vi "ProcessTemplate (Minimal).vi"   [LabVIEW 2021]
uses:
  SMO/SMO.lvclass
types:
  T1 = typedef "smo.lvlib/SMO.lvclass/Protected Events.ctl" = cluster{"StopProcesses":refnum<user-event>, "AbortProcesses":refnum<user-event>, "Config Changed":refnum<user-event>, "Dependency":refnum<user-event>}
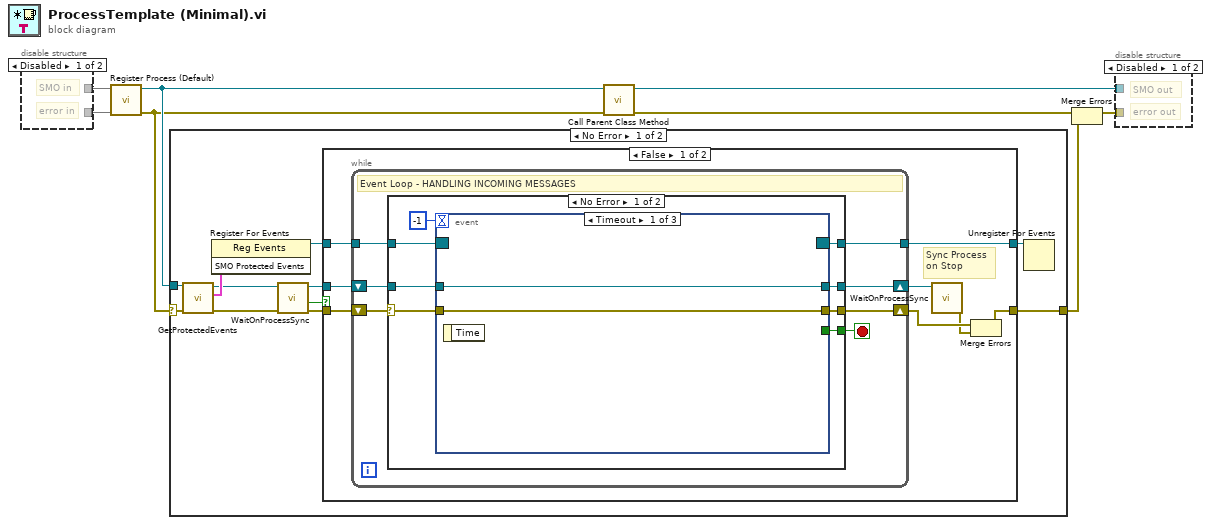
[diagram p0: block diagram]
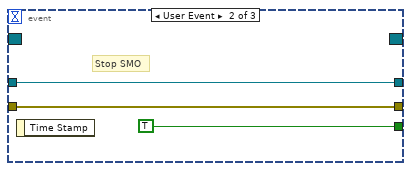
[diagram p4: hidden frame]
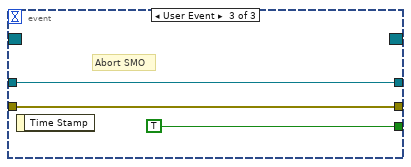
[diagram p5: hidden frame]
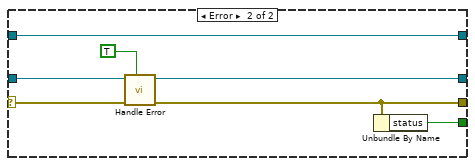
[diagram p6: hidden frame]
diagram:
  n1 = disable-structure shown="Disabled" {
    disable-tunnel: [_ _] -> w2
    disable-tunnel: [_ _] -> w1
    frame Disabled {
      # "error in"
      # "SMO in"
    }
    frame Enabled {
    }
  }
  n2 = call "Register Process (Default).vi"("error in (no error)"=w1, "SMO"=w2) -> ("error out"=w3:errorcluster, "SelfRef"=w4:refnum<class "SMO.lvclass">)  [unwired: 8 in]
  n3 = case shown="No Error" w3 {
    selector: w3 -> [w15 w60]
    tunnel: w4 -> [w18 _]
    tunnel: [w11 w60] -> w7
    frame No Error {
      n4 = call "GetProtectedEvents.vi"("error in (no error)"=w15, "SMO"=w18) -> ("error out"=w16:errorcluster, "SMO Protected Events"=w19:T1, "SMO out"=w17:refnum<class "SMO.lvclass">)  [unwired: 7 in]
      n5 = register-events(w19) -> (reference out=w9:refnum<event-registration>)  [unwired: 2 in, 1 out]
      n6 = call "WaitOnProcessSync.vi"("error in (no error)"=w16, "SMO"=w17) -> ("error out"=w13:errorcluster, "Don't run?"=w12:bool, "SMO out"=w14:refnum<class "SMO.lvclass">)  [unwired: 7 in]
      n7 = case shown="False" w12 {
        tunnel: w13 -> [w23 w58]
        tunnel: w14 -> [w25 _]
        tunnel: w9 -> [w27 w59]
        tunnel: [w20 w58] -> w11
        tunnel: [w26 w59] -> w10
        frame False {
          # "Sync Process\non Stop"
          n8 = while {
            tunnel: w27 -> [w34]
            tunnel: [w33] -> w26
            shift-right: [w30] -> w24
            shift-left: w25 -> [w31]
            shift-right: [w29] -> w22
            shift-left: w23 -> [w28]
            stop <- w32 stop-if-true
            # "Event Loop - HANDLING INCOMING MESSAGES"
            n9 = case shown="No Error" w28 {
              selector: w28 -> [w35 w55]
              tunnel: w34 -> [w41 w57]
              tunnel: [w40 w57] -> w33
              tunnel: [w39 w51] -> w32
              tunnel: w31 -> [w38 w54]
              tunnel: [w37 w53] -> w30
              tunnel: [w36 w52] -> w29
              frame No Error {
                n10 = event shown="[0] Timeout" {
                  selector: w41 -> [_ _ _]
                  dyn-events: [_ _ _] -> w40
                  timeout: -1 -> [_ _ _]
                  tunnel: [_ TRUE TRUE] -> w39
                  tunnel: w38 -> [w44 w46 w49]
                  tunnel: [w44 w46 w49] -> w37
                  tunnel: [w43 w45 w48] -> w36
                  tunnel: w35 -> [w43 w45 w48]
                  event Timeout {
                    n11 = event-data() -> ()  [unwired: 1 in, 1 out]
                  }
                  event User Event {
                    # "Stop SMO"
                    n12 = event-data() -> ()  [unwired: 1 in, 1 out]
                  }
                  event User Event {
                    # "Abort SMO"
                    n13 = event-data() -> ()  [unwired: 1 in, 1 out]
                  }
                }
              }
              frame Error {
                n14 = call-dynamic "Handle Error.vi"("Stop on Unhandled Error (T)"=TRUE, "error in"=w55, "SMO"=w54) -> ("handling error"=w52:errorcluster, "SMO out"=w53:refnum<class "SMO.lvclass">)  [unwired: 6 in, 1 out]
                n15 = Unbundle By Name(w52) -> ("status"=w51:bool)
              }
            }
          }
          n16 = call "WaitOnProcessSync.vi"("SMO"=w24) -> ("error out"=w21:errorcluster)  [unwired: 8 in, 2 out]
          n17 = Merge Errors(w22, w21) -> (w20:errorcluster)
        }
        frame True {
        }
      }
      n18 = Unregister For Events(event registration refnum=w10) -> ()  [unwired: 1 in, 1 out]
    }
    frame Error {
    }
  }
  n19 = call-parent "Call Parent Class Method"("error in"=w3, "SMO"=w4) -> ("error out"=w8:errorcluster, "SMO out"=w5:refnum<class "SMO.UI.lvclass">)  [unwired: 8 in]
  n20 = Merge Errors(w8, w7) -> (w6:errorcluster)
  n21 = disable-structure shown="Disabled" {
    disable-tunnel: w6 -> [_ _]
    disable-tunnel: w5 -> [_ _]
    frame Disabled {
      # "error out"
      # "SMO out"
    }
    frame Enabled {
    }
  }
